vi "Match Pattern.vi"(4 "Before Match":refnum<class "Abs_String.lvclass">, 5 "Offset Past Match":refnum<class "Abs_I32 Integer.lvclass">, 6 "After Match":refnum<class "Abs_String.lvclass">, 7 "Match":refnum<class "Abs_String.lvclass">, 9 "Offset":i32, 10 "Pattern":string, 11 "String":T1) -> (3 "Result":refnum<class "MatchPattern_STR.lvclass">)   [LabVIEW 2021]
uses:
  Support/Compare/One Term/STR/Support/Abstract Type.ctl
  Abs_Types/String/Abs_String.lvclass
  Support/Match Pattern/MatchPattern_STR.lvclass
  C:/TSA/LV_Abstract/Source/Functions/Support/Compare/One Term/STR/AbsComp_One Term_STR.lvclass
  Abs_Types/I32 Integer/Abs_I32 Integer.lvclass
  Support/Compare/One Term/STR/AbsComp_One Term_STR.lvclass/AbsComp_One Term_STR.ctl
  Support/Match Pattern/MatchPattern_STR.lvclass/MatchPattern_STR.ctl
  Support/Compare/One Term/STR/Properties/Write String A.vi
  Support/Match Pattern/Properties/Write Pattern.vi
  Support/Match Pattern/Properties/Write Offset.vi
  Support/Match Pattern/Properties/Write Offset Past Match.vi
  Support/Match Pattern/Properties/Write Match.vi
  Support/Match Pattern/Properties/Write After Match.vi
  Support/Match Pattern/Properties/Write Before Match.vi
  Support/Compare/One Term/STR/AbsComp_One Term_STR.lvclass
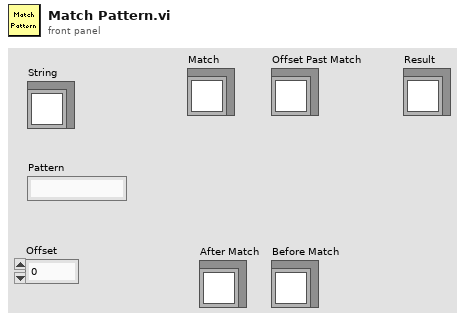
[diagram p1: front panel]
types:
  T1 = typedef "AbsComp_One Term_STR.lvclass/Abstract Type.ctl" = refnum<class "Abs_String.lvclass">
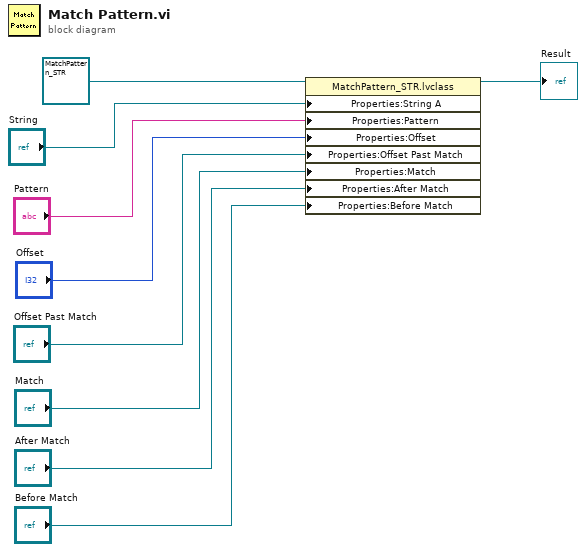
[diagram p0: block diagram]
diagram:
  n1 = property class="MatchPattern_STR.lvclass"(reference=refnum<class "MatchPattern_STR.lvclass"> refnum ("MatchPattern_STR.lvclass"), "Properties:String A"="String", "Properties:Pattern"="Pattern", "Properties:Offset"="Offset", "Properties:Offset Past Match"="Offset Past Match", "Properties:Match"="Match", "Properties:After Match"="After Match", "Properties:Before Match"="Before Match") -> (reference out=→"Result":refnum<class "MatchPattern_STR.lvclass">)  [unwired: 1 in, 1 out]
